vi "GetError.vi"(7 "DLLFunction":string, 8 "error in":errorcluster, 11 "code":i32) -> (0 "error out":errorcluster)   [LabVIEW 2022 SP3, in "EClib functions.lvlib"]
uses:
  EClib functions.lvlib
  <vilib>/Utility/error.llb/Trim Whitespace One-Sided.vi
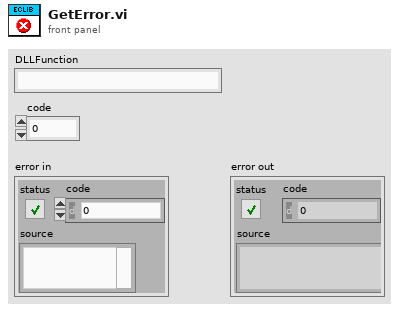
[diagram p1: front panel]
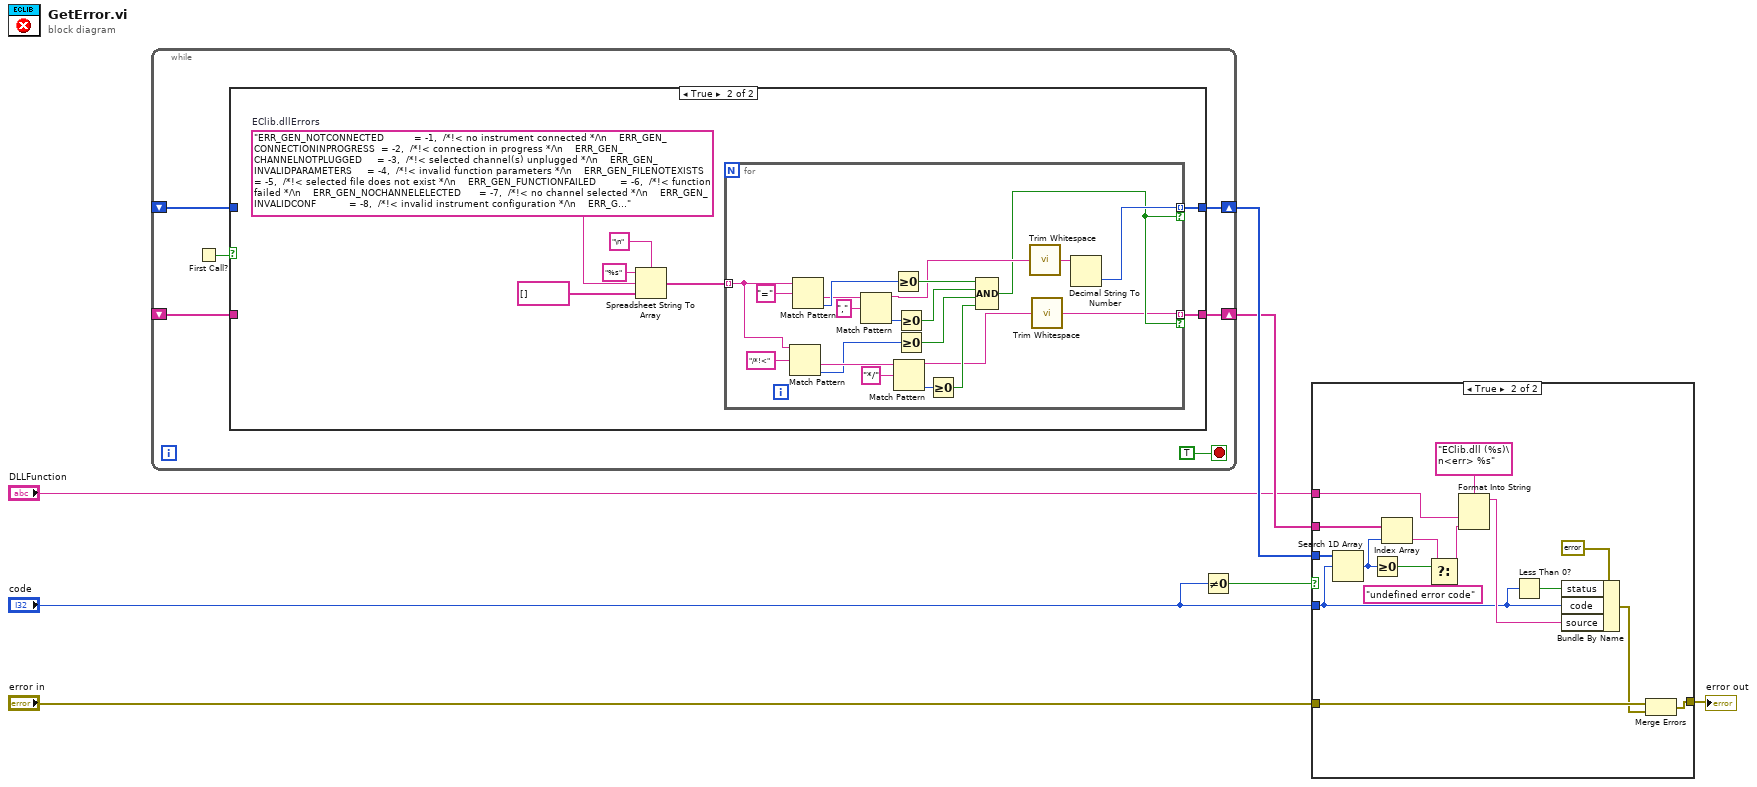
[diagram p0: block diagram]
diagram:
  n1 = while {
    shift-right: [w13] -> w7
    shift-left: _ -> [w9]
    shift-right: [w12] -> w6
    shift-left: _ -> [w8]
    stop <- TRUE stop-if-true
    n2 = First Call?() -> (First Call?: T/F=w10:bool)
    n3 = case shown="True" w10 {
      tunnel: [w15 w17] -> w13
      tunnel: [w14 w16] -> w12
      tunnel: w9 -> [w15 _]
      tunnel: w8 -> [w14 _]
      frame False {
      }
      frame True {
        w22 = "ERR_GEN_NOTCONNECTED          = -1,  /*!< no instrument connected */\n    ERR_GEN_CONNECTIONINPROGRESS  = -2,  /*!< connection in progress */\n    ERR_GEN_CHANNELNOTPLUGGED     = -3,  /*!< selected channel(s) unplugged */\n    ERR_GEN_INVALIDPARAMETERS     = -4,  /*!< invalid function parameters */\n    ERR_GEN_FILENOTEXISTS         = -5,  /*!< selected file does not exist */\n    ERR_GEN_FUNCTIONFAILED        = -6,  /*!< function failed */\n    ERR_GEN_NOCHANNELELECTED      = -7,  /*!< no channel selected */\n    ERR_GEN_INVALIDCONF           = -8,  /*!< invalid instrument configuration */\n    ERR_GEN_ECLAB_LOADED          = -9,  /*!< EC-Lab firmware loaded on the instrument */\n    ERR_GEN_LIBNOTCORRECTLYLOADED = -10, /*!< library not correctly loaded in memory */\n    ERR_GEN_USBLIBRARYERROR       = -11, /*!< USB library not correctly loaded in memory */\n    ERR_GEN_FUNCTIONINPROGRESS    = -12, /*!< function of the library already in progress */\n    ERR_GEN_CHANNEL_RUNNING       = -13, /*!< selected channel(s) already used */\n    ERR_GEN_DEVICE_NOTALLOWED     = -14, /*!< device not allowed */\n    ERR_GEN_UPDATEPARAMETERS      = -15, /*!< Invalid update function parameters */\n \n    /* Instrument error codes */\n    ERR_INSTR_VMEERROR        = -101, /*!< internal instrument communication failed */\n    ERR_INSTR_TOOMANYDATA     = -102, /*!< too many data to transfer from the instrument (device error) */\n    ERR_INSTR_RESPNOTPOSSIBLE = -103, /*!< selected channel(s) unplugged (device error) */\n    ERR_INSTR_RESPERROR       = -104, /*!< instrument response error */\n    ERR_INSTR_MSGSIZEERROR    = -105, /*!< invalid message size */\n \n    /* Communication error codes */\n    ERR_COMM_COMMFAILED         = -200, /*!< communication failed with the instrument */\n    ERR_COMM_CONNECTIONFAILED   = -201, /*!< cannot establish connection with the instrument */\n    ERR_COMM_WAITINGACK         = -202, /*!< waiting for the instrument response */\n    ERR_COMM_INVALIDIPADDRESS   = -203, /*!< invalid IP address */\n    ERR_COMM_ALLOCMEMFAILED     = -204, /*!< cannot allocate memory in the instrument */\n    ERR_COMM_LOADFIRMWAREFAILED = -205, /*!< cannot load firmware into selected channel(s) */\n    ERR_COMM_INCOMPATIBLESERVER = -206, /*!< communication firmware not compatible with the library */\n    ERR_COMM_MAXCONNREACHED     = -207, /*!< maximum number of allowed connections reached */\n \n    /* Firmware error codes */\n    ERR_FIRM_FIRMFILENOTEXISTS    = -300, /*!< cannot find kernel.bin file */\n    ERR_FIRM_FIRMFILEACCESSFAILED = -301, /*!< cannot read kernel.bin file */\n    ERR_FIRM_FIRMINVALIDFILE      = -302, /*!< invalid kernel.bin file */\n    ERR_FIRM_FIRMLOADINGFAILED    = -303, /*!< cannot load kernel.bin on the selected channel(s) */\n    ERR_FIRM_XILFILENOTEXISTS     = -304, /*!< cannot find x100_01.txt file */\n    ERR_FIRM_XILFILEACCESSFAILED  = -305, /*!< cannot read x100_01.txt file */\n    ERR_FIRM_XILINVALIDFILE       = -306, /*!< invalid x100_01.txt file */\n    ERR_FIRM_XILLOADINGFAILED     = -307, /*!< cannot load x100_01.txt file on the selected channel(s) */\n    ERR_FIRM_FIRMWARENOTLOADED    = -308, /*!< no firmware loaded on the selected channel(s) */\n    ERR_FIRM_FIRMWAREINCOMPATIBLE = -309, /*!< loaded firmware not compatible with the library */\n \n    /* Technique error codes */\n    ERR_TECH_ECCFILENOTEXISTS    = -400, /*!< cannot find the selected ECC file */\n    ERR_TECH_INCOMPATIBLEECC     = -401, /*!< ECC file not compatible with the channel firmware */\n    ERR_TECH_ECCFILECORRUPTED    = -402, /*!< ECC file corrupted */\n    ERR_TECH_LOADTECHNIQUEFAILED = -403, /*!< cannot load the ECC file */\n    ERR_TECH_DATACORRUPTED       = -404, /*!< data returned by the instrument are corrupted */\n    ERR_TECH_MEMFULL             = -405,  /*!< cannot load techniques: full memory */"  # EClib.dllErrors
        n4 = Spreadsheet String To Array(delimiter (Tab)="\n", format string="%s", spreadsheet string=w22, array type (2D Dbl)=string[] []) -> (array=w18:string[])
        n5 = for {
          tunnel: w18 -> [w40] mode=indexing
          tunnel: [w27] -> w17 mode=indexing if=w25
          tunnel: [w23] -> w16 mode=indexing if=w25
          n6 = Match Pattern(string=w40, regular expression="/*!<") -> (after substring=w34:string, offset past match=w32:i32)  [unwired: 1 in, 2 out]
          n7 = Match Pattern(string=w40, regular expression="=") -> (after substring=w39:string, offset past match=w42:i32)  [unwired: 1 in, 2 out]
          n8 = Match Pattern(string=w39, regular expression=",") -> (before substring=w28:string, offset past match=w37:i32)  [unwired: 1 in, 2 out]
          n9 = Greater Or Equal To 0?(x=w42) -> (x >= 0?=w36:bool)
          n10 = Match Pattern(string=w34, regular expression="*/") -> (before substring=w26:string, offset past match=w30:i32)  [unwired: 1 in, 2 out]
          n11 = Greater Or Equal To 0?(x=w37) -> (x >= 0?=w35:bool)
          n12 = Greater Or Equal To 0?(x=w32) -> (x >= 0?=w31:bool)
          n13 = Greater Or Equal To 0?(x=w30) -> (x >= 0?=w29:bool)
          n14 = Compound Arithmetic op=AND(w36, w35, w31, w29) -> (w25:bool)
          n15 = call <vilib>:"Trim Whitespace.vi"("string"=w28) -> ("trimmed string"=w24:string)  [unwired: 1 in]
          n16 = call <vilib>:"Trim Whitespace.vi"("string"=w26) -> ("trimmed string"=w23:string)  [unwired: 1 in]
          n17 = Decimal String To Number(string=w24) -> (number=w27:i32)  [unwired: 2 in, 1 out]
        }
      }
    }
  }
  n18 = Not Equal To 0?(x="code") -> (x != 0?=w3:bool)
  n19 = case shown="True" w3 {
    tunnel: w7 -> [_ w59]
    tunnel: w6 -> [_ w57]
    tunnel: [w44 w49] -> w5
    tunnel: "code" -> [_ w46]
    tunnel: "error in" -> [w44 w51]
    tunnel: "DLLFunction" -> [_ w47]
    frame False {
    }
    frame True {
      n20 = Search 1D Array(1D array=w59, element=w46) -> (index of element=w52:i32)  [unwired: 1 in]
      n21 = Greater Or Equal To 0?(x=w52) -> (x >= 0?=w58:bool)
      n22 = Index Array(array=w57, index=w52) -> (element=w56:string)
      n23 = Select(t=w56, s=w58, f="undefined error code") -> (s? t:f=w48:string)
      n24 = Format Into String(format string="EClib.dll (%s)\n<err> %s", w47, w48) -> (resulting string=w53:string)  [unwired: 2 in, 1 out]
      n25 = Less Than 0?(x=w46) -> (x < 0?=w45:bool)
      n26 = Bundle By Name(cluster=errorcluster {"status"=TRUE, "code"=0, "source"=""} ("error out"), "status"=w45, "code"=w46, "source"=w53) -> (w50:errorcluster)
      n27 = Merge Errors(w51, w50) -> (w49:errorcluster)
    }
  }
  "error out" <- w5
